vi "Serialize Connection Info.vi"(7 "Field Delimiter (::)":string="::", 8 "error in (no error)":errorcluster, 11 "Connection Info":T1) -> (0 "error out 2":errorcluster, 3 "Serialized Connection Info":string)   [LabVIEW 2020, in "plugin_flodx_ph_probe.lvlib" / "plugin.lvlib" / "Instrument Manager.lvlib"]
doc: "Serializes the connection info. By default, it serializes to the string \"<visa_resource>::<pump_address>\"."
uses:
  Instrument Manager.lvlib
  Connection Info.ctl
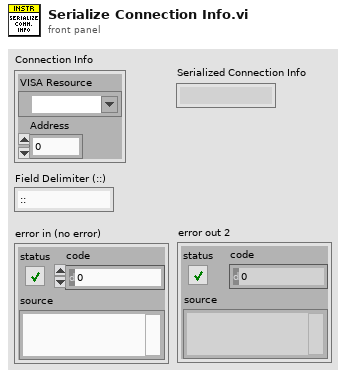
[diagram p1: front panel]
types:
  T1 = typedef "plugin_flodx_ph_probe.lvlib/plugin.lvlib/Instrument Manager.lvlib/Connection Info.ctl" = cluster{"VISA Resource":refnum<visa-resource-name>, "Address":u8}
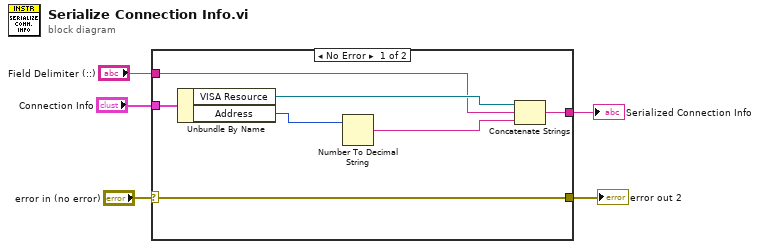
[diagram p0: block diagram]
diagram:
  n1 = case shown="No Error" "error in (no error)" {
    selector: "error in (no error)" -> [w12 w14]
    tunnel: [w12 w14] -> w4
    tunnel: "Connection Info" -> [w11 _]
    tunnel: "Field Delimiter (::)" -> [w6 _]
    tunnel: [w10 ""] -> w2
    frame No Error {
      n2 = Unbundle By Name(w11) -> ("VISA Resource"=w9:refnum<visa-resource-name>, "Address"=w8:u8)
      n3 = Number To Decimal String(number=w8) -> (decimal integer string=w7:string)  [unwired: 1 in]
      n4 = Concatenate Strings(w9, w6, w7) -> (w10:string)
    }
    frame Error {
    }
  }
  "error out 2" <- w4
  "Serialized Connection Info" <- w2
